vi "Gain.vi"(6 "DMM VISA in":refnum<visa-resource-name>, 7 "HMF VISA in":refnum<visa-resource-name>, 8 "error in (no error)":errorcluster {"code" format="%.0x"}, 9 "R":dbl, 10 "L":dbl, 11 "Max v input":dbl) -> (0 "error out":errorcluster {"code" format="%.0x"}, 3 "Polynomial coeff":dbl[](array[numeric]), 4 "DMM VISA out":refnum<visa-resource-name>, 5 "HMF VISA out":refnum<visa-resource-name>)   [LabVIEW 2015]
uses:
  <vilib>/express/express arith-compare/Formula/XNode/ExpressFormulaBlockNode.xnode
  <vilib>/Analysis/NI_AALPro.lvlib
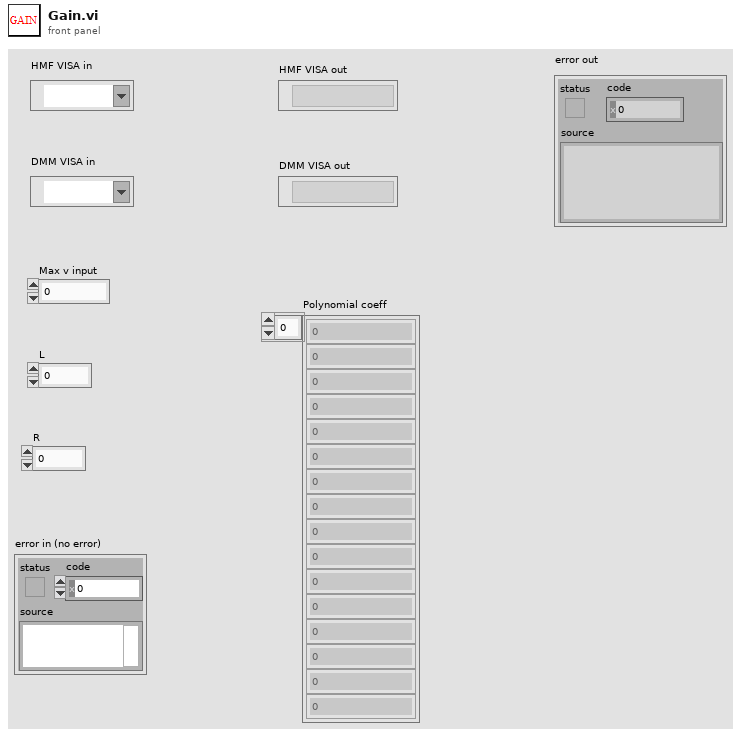
[diagram p1: front panel]
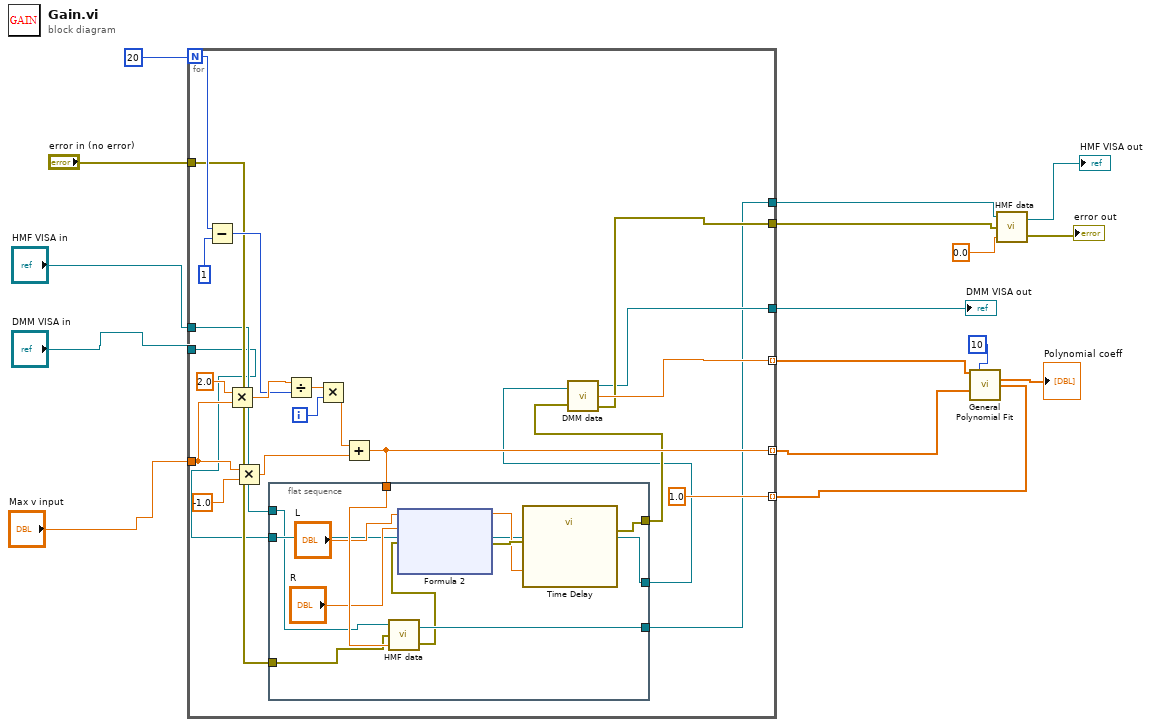
[diagram p0: block diagram]
diagram:
  n1 = for {
    N: 20 -> [w33]
    tunnel: "Max v input" -> [w36]
    tunnel: [w23] -> w9 mode=indexing
    tunnel: [w26] -> w10 mode=indexing
    tunnel: "DMM VISA in" -> [w18]
    tunnel: "HMF VISA in" -> [w20]
    tunnel: [1.0] -> w8 mode=indexing
    tunnel: [w24] -> w14
    tunnel: [w25] -> w12
    tunnel: "error in (no error)" -> [w22]
    tunnel: [w19] -> w1
    i -> [w29]
    n2 = Subtract(x=w33, y=1) -> (x-y=w31:i32)
    n3 = Multiply(x=2.0, y=w36) -> (x*y=w34:dbl)
    n4 = Multiply(x=w36, y=-1.0) -> (x*y=w37:ext)
    n5 = flat-sequence {
      tunnel: w23 -> [w47]
      tunnel: w22 -> [w42]
      tunnel: [w44] -> w21
      tunnel: w20 -> [w39]
      tunnel: [w43] -> w19
      tunnel: w18 -> [w40]
      tunnel: [w40] -> w17
      frame #0 {
        n6 = call "HMF data.vi"("DC offset"=w47, "error in (no error)"=w42, "VISA resource name"=w39) -> ("error out"=w41:errorcluster, "VISA resource name out"=w43:refnum<visa-resource-name>)
        n7 = xnode "Formula 2"("X1"="L", "X2"="R", "error in (no error)"=w41) -> ("Result"=w48:dbl, "error out"=w49:errorcluster)
        n8 = call "Time Delay"("error in (no error)"=w49, "Delay Time (s)"=w48) -> ("error out"=w44:errorcluster)  [unwired: 9 in]
      }
    }
    n9 = Divide(x=w34, y=w31) -> (x/y=w30:ext)
    n10 = Multiply(x=w30, y=w29) -> (x*y=w28:ext)
    n11 = Add(x=w28, y=w37) -> (x+y=w23:ext)
    n12 = call "DMM data.vi"("VISA resource name"=w17, "error in (no error)"=w21) -> ("VISA resource name out"=w24:refnum<visa-resource-name>, "Voltage"=w26:dbl, "error out"=w25:errorcluster)
  }
  "DMM VISA out" <- w14
  n13 = call <vilib>:"General Polynomial Fit.vi"("Y"=w10, "polynomial order"=10, "X"=w9, "Weight"=w8) -> ("Polynomial Coefficients"=→"Polynomial coeff":dbl[])  [unwired: 8 in, 3 out]
  n14 = call "HMF data.vi"("DC offset"=0.0, "error in (no error)"=w12, "VISA resource name"=w1) -> ("error out"=→"error out":errorcluster, "VISA resource name out"=→"HMF VISA out":refnum<visa-resource-name>)
